vi "HDBn.vi"(1 "输入":i8[](array[numeric]), 2 "n":dbl=3.0) -> (0 "输出":i8[](array[numeric]))   [LabVIEW 2018]
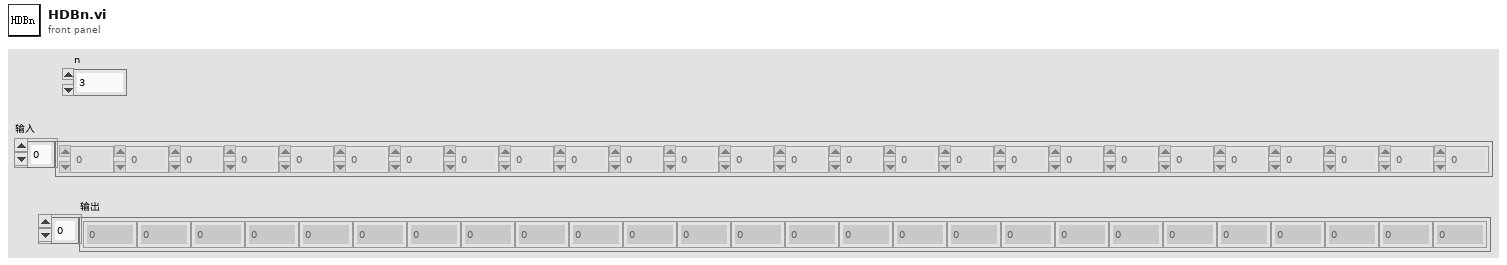
[diagram p1: front panel]
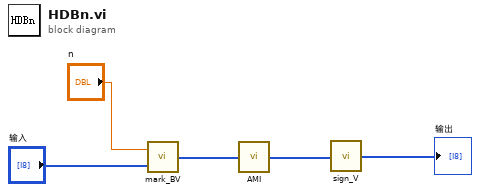
[diagram p0: block diagram]
diagram:
  n1 = call "mark_BV.vi"("输入"="输入", "n"="n") -> ("输出"=w3:i8[])
  n2 = call "AMI.vi"("输入"=w3) -> ("输出"=w2:i8[])
  n3 = call "sign_V.vi"("输入"=w2) -> ("输出"=→"输出":i8[])
